vi "events.vi"() -> ()   [LabVIEW 2013]
uses:
  domain.ctl
  protocol.ctl
  lvnano.lvlib
  lvnanomsg.dll
panel:
  in  "stop":bool
  out "msg in":string
  in  "msg out":string
  in  "send":bool
  in  "messages":i32=1
  out "error out":errorcluster
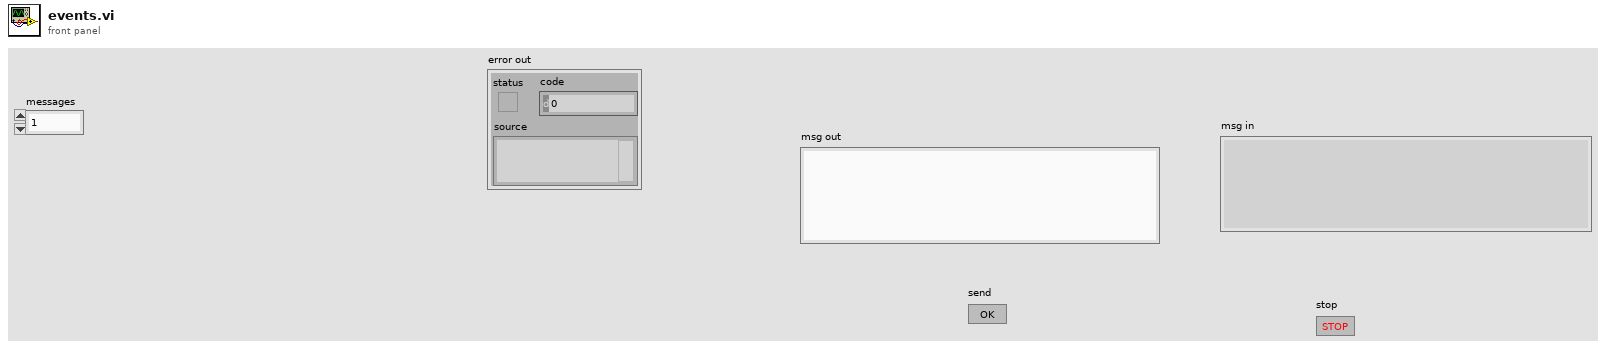
[diagram p1: front panel]
types:
  T1 = typedef "lvnano.lvlib/protocol.ctl" = i32
  T2 = typedef "lvnano.lvlib/domain.ctl" = enum16{"Invalid", "AF_SP", "AF_SP_RAW"}
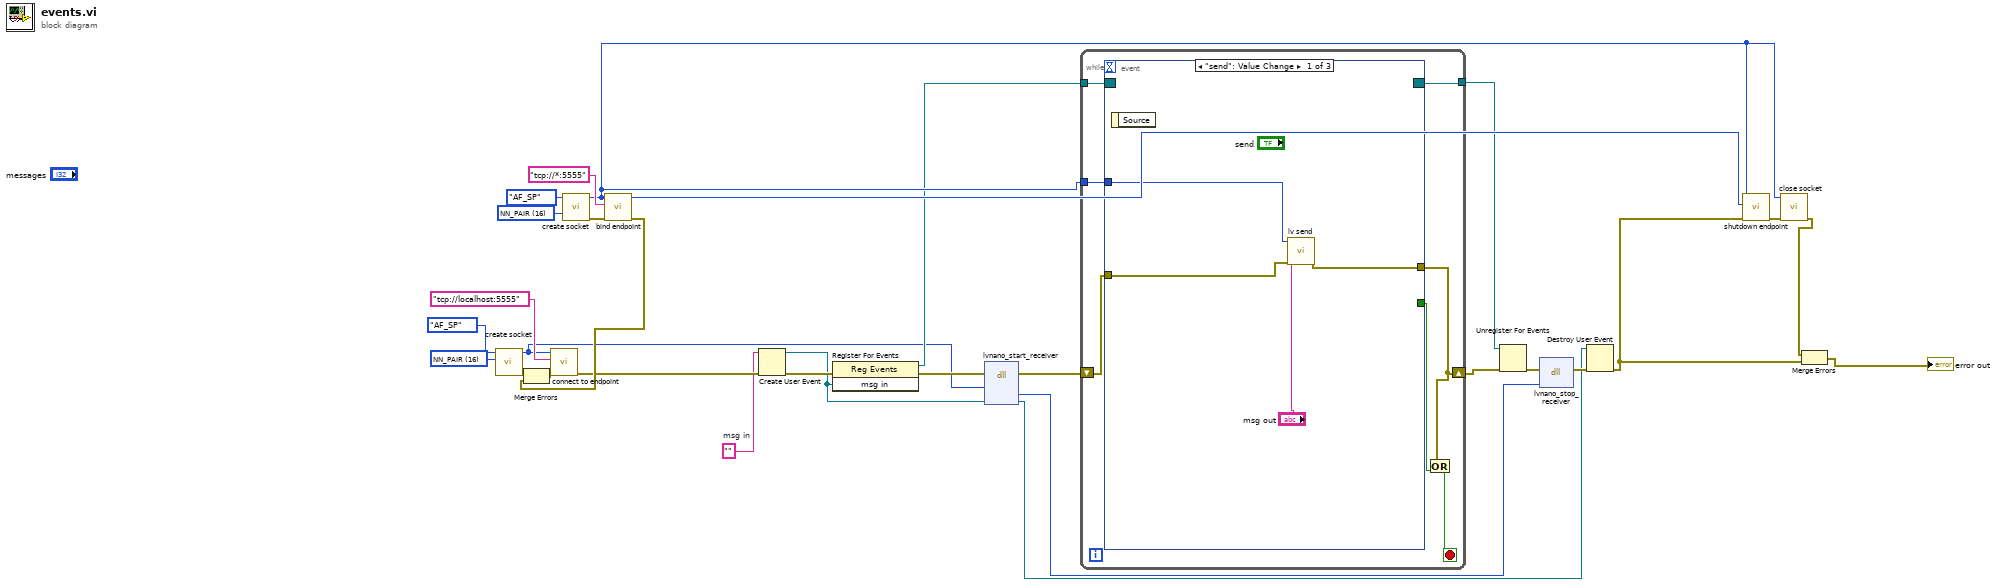
[diagram p0: block diagram]
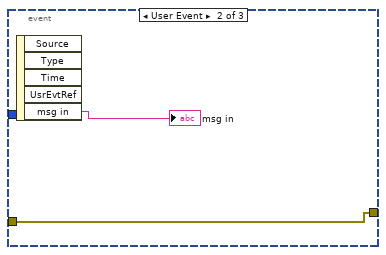
[diagram p2: hidden frame]
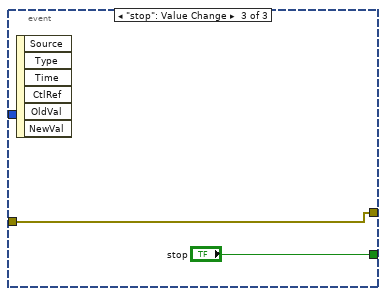
[diagram p3: hidden frame]
diagram:
  w12 = ""  # msg in
  w17 = T1 16 items=["NN_PUSH"=80, "NN_PULL"=81, "NN_BUS"=112, "NN_PAIR"=16, "NN_PUB"=32, "NN_SUB"=33, "NN_REQ"=48, "NN_REP"=49, "NN_SURVEYOR"=96, "NN_RESPONDENT"=97] ("protocol")
  w18 = T1 16 items=["NN_PUSH"=80, "NN_PULL"=81, "NN_BUS"=112, "NN_PAIR"=16, "NN_PUB"=32, "NN_SUB"=33, "NN_REQ"=48, "NN_REP"=49, "NN_SURVEYOR"=96, "NN_RESPONDENT"=97] ("protocol")
  n1 = call "create socket.vi"("protocol"=w17, "domain"=domain."AF_SP") -> ("error out"=w25:errorcluster, "socket"=w1:i64)  [unwired: 8 in]
  n2 = call "create socket.vi"("protocol"=w18, "domain"=domain."AF_SP") -> ("error out"=w29:errorcluster, "socket"=w14:i64)  [unwired: 8 in]
  n3 = call "bind endpoint.vi"("error in"=w29, "address"="tcp://*:5555" ("addr"), "socket"=w14) -> ("error out"=w19:errorcluster, "endpoint"=w21:i32)  [unwired: 7 in]
  n4 = Merge Errors(w25, w19) -> (w20:errorcluster)
  n5 = call "connect to endpoint.vi"("error in"=w20, "address"="tcp://localhost:5555" ("addr"), "socket"=w1) -> ("error out"=w16:errorcluster)  [unwired: 7 in, 1 out]
  n6 = Create User Event(user event datatype=w12, error in=w16) -> (user event=w4:refnum<user-event>, error out=w13:errorcluster)
  n7 = register-events(error in=w13, w4) -> (reference out=w10:refnum<event-registration>, error out=w11:errorcluster)  [unwired: 1 in]
  n8 = dll-call lib="C:/Users/Daniel/Documents/nanomsg/lvnano/lvnanomsg.*" fn="lvnano_start_receiver"(error in=w11, "s"=w1, "event"=w4) -> (error out=w6:errorcluster, "rthread context pointer"=w2:i64, "event"=w3:refnum<user-event>)  [unwired: 5 in, 1 out]
  n9 = while {
    shift-right: [w35] -> w15
    shift-left: w6 -> [w36]
    tunnel: w14 -> [w37]
    tunnel: w10 -> [w34]
    tunnel: [w33] -> w8
    stop <- w32 stop-if-true
    n10 = event shown="[0] \"send\": Value Change" {
      selector: w34 -> [_ _ _]
      dyn-events: [_ _ _] -> w33
      timeout: _ -> [_ _ _]
      tunnel: w37 -> [w41 _ _]
      tunnel: w36 -> [w39 w42 w44]
      tunnel: [w38 w42 w44] -> w35
      tunnel: [_ _ "stop"] -> w31
      event "send": Value Change {
        n11 = event-data() -> ()  [unwired: 1 in, 1 out]
        n12 = call "lv send.vi"("error in"=w39, "data"="msg out", "socket"=w41) -> ("error out"=w38:errorcluster)  [unwired: 8 in]
      }
      event User Event {
        n13 = event-data() -> ("msg in"=→"msg in":string)  [unwired: 1 in, 4 out]
      }
      event "stop": Value Change {
        n14 = event-data() -> ()  [unwired: 1 in, 6 out]
      }
    }
    n15 = Or(x=w35, y=w31) -> (x .or. y?=w32:bool)
  }
  n16 = Unregister For Events(event registration refnum=w8, error in=w15) -> (error out=w9:errorcluster)
  n17 = dll-call lib="C:/Users/Daniel/Documents/nanomsg/lvnano/lvnanomsg.dll" fn="lvnano_stop_receiver"(error in=w9, "rthread context"=w2) -> (error out=w5:errorcluster)  [unwired: 4 in, 1 out]
  n18 = Destroy User Event(user event=w3, error in=w5) -> (error out=w7:errorcluster)
  n19 = call "shutdown endpoint.vi"("error in"=w7, "endpoint"=w21, "socket"=w14) -> ("error out"=w23:errorcluster)  [unwired: 8 in]
  n20 = call "close socket.vi"("error in"=w23, "socket"=w14) -> ("error out"=w22:errorcluster)  [unwired: 9 in]
  n21 = Merge Errors(w22, w7) -> (→"error out":errorcluster)
